vi "FR Estimate measurement time.vi"(11 "FFmeter settings":T1={"AC Source"={"AC Source type"=enum."Fluke 5XXX calibrator", "VISA"="", "Ref. clock (Hz)"=0.0, "status ref"=refnum}, "TWM pipe"="\\\\.\\pipe\\TWM:server", "Measurement status ref"=refnum, "TWM Status ref"=refnum, "Abort ref"=refnum, "DC meter"={"DC meter type"=enum."H/A/K 3458", "DC meter VISA"="", "NPLC"=10, "status ref"=refnum}, "FR Measurement properties"={"Measurement frequencies (Hz)"=[1000.0], "Sampling frequency (Hz)"=500000.0, "Signal amplitude (V)"=4.5, "AC-DC settle time (s)"=20.0, "Record length (multiples of period)"=[1000.0, 10000.0, 1000.0], "Measurement template file"=path "", "Row of START keyword"=1, "Row of STOP keyword"=0, "Calculate RMS from samples"=FALSE, "AC-DC warm up time (s)"=300.0, "Measurement template line"=[], "DC meter readings No."=10, "Algorithm"="TWM-WFFT", "Simultaneous measurement"=FALSE}, "Skip waiting ref"=refnum, "Octave paths"={"GNU Octave path"=path "C:/Program Files/GNU Octave/Octave-6.2.0/mingw64/bin", "TWM+QWTB path"=path "C:/Users/labina/Desktop/TWM-1.8.7.0-full/octprog", "lvlib path"=path "D:/martin/WAC/WACsw - github/control_software/Filter function meter/external libraries/GOLPI 0.7.3.1 source distribution LV 20.0 32 bit/lv_proc.dll"}, "FR Template definition"={"Keywords column"=0, "Sig. freq. column"=1, "Rec. len. column"=2, "Meas. points. row min to read"=9, "Meas. points. row max to read"=1509, "Properties column"=4, "Properties row start"=1, "Properties row end"=5, "Keyword START regexp"="", "Keyword STOP regexp"="", "HW data column"=7, "HW data row start"=1, "HW data row end"=3, "TIme and date column start"=3, "Digitizer value column start "=4, "DC mean column start "=6, "DC readings column start"=10}, "Recalculate-skip already calculated"=FALSE} {"FR Measurement properties"."Record length (multiples of period)" format="%#_3p"; "FR Measurement properties"."Sampling frequency (Hz)" format="%#_3p"; "FR Measurement properties"."Measurement frequencies (Hz)" format="%#_3p"}) -> (1 "Estimate as formatted text":string, 3 "Estimate of measurement time (s)":dbl)   [LabVIEW 2020]
doc: "Estimates the total measurement time based on the measurement settings and devices settings."
uses:
  FR GUI/Type definitions/FRmeter settings.ctl
  General AC source/Type definitions/AC Source.ctl
  General AC source/Type definitions/AC Source type.ctl
  General DC meter/Type definitions/DC meter.ctl
  General DC meter/Type definitions/DC meter type.ctl
  FR Measurement/Type definitions/FR Measuement properties.ctl
  Type definitions/FR Template definition.ctl
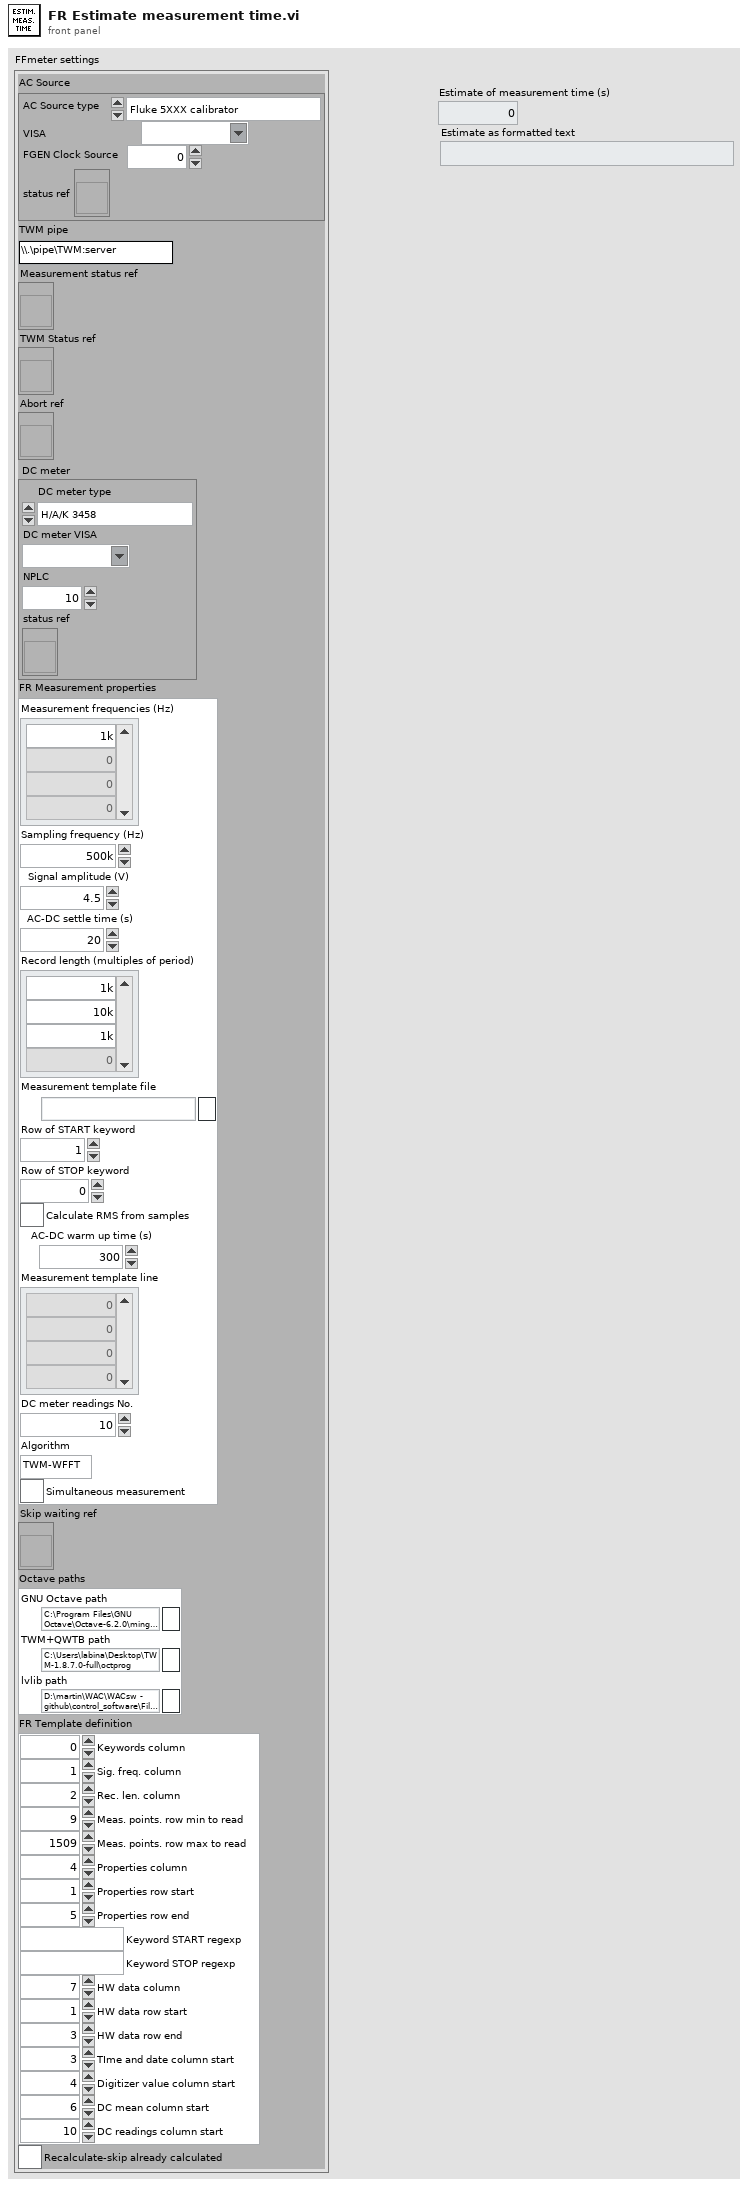
[diagram p1: front panel]
types:
  T1 = typedef "FRmeter settings.ctl" = cluster{"AC Source":T2, "TWM pipe":string, "Measurement status ref":refnum<vi>, "TWM Status ref":refnum<vi>, "Abort ref":refnum<vi>, "DC meter":T4, "FR Measurement properties":T6, "Skip waiting ref":refnum<vi>, "Octave paths":cluster{"GNU Octave path":path, "TWM+QWTB path":path, "lvlib path":path}, "FR Template definition":T7, "Recalculate-skip already calculated":bool}
  T2 = typedef "AC Source.ctl" = cluster{"AC Source type":T3, "VISA":refnum<visa-resource-name>, "Ref. clock (Hz)":dbl, "status ref":refnum<vi>}
  T3 = typedef "AC Source type.ctl" = enum16{"Fluke 5XXX calibrator", "Tektronix AFG3000 series", "dummy"}
  T4 = typedef "DC meter.ctl" = cluster{"DC meter type":T5, "DC meter VISA":refnum<visa-resource-name>, "NPLC":i32, "status ref":refnum<vi>}
  T5 = typedef "DC meter type.ctl" = enum16{"H/A/K 3458", "Fluke 8508A", "dummy", "Keithley 2182"}
  T6 = typedef "FR Measuement properties.ctl" = cluster{"Measurement frequencies (Hz)":dbl[], "Sampling frequency (Hz)":dbl, "Signal amplitude (V)":dbl, "AC-DC settle time (s)":dbl, "Record length (multiples of period)":dbl[], "Measurement template file":path, "Row of START keyword":i32, "Row of STOP keyword":i32, "Calculate RMS from samples":bool, "AC-DC warm up time (s)":dbl, "Measurement template line":i32[], "DC meter readings No.":i32, "Algorithm":string, "Simultaneous measurement":bool}
  T7 = typedef "FR Template definition.ctl" = cluster{"Keywords column":i32, "Sig. freq. column":i32, "Rec. len. column":i32, "Meas. points. row min to read":i32, "Meas. points. row max to read":i32, "Properties column":i32, "Properties row start":i32, "Properties row end":i32, "Keyword START regexp":string, "Keyword STOP regexp":string, "HW data column":i32, "HW data row start":i32, "HW data row end":i32, "TIme and date column start":i32, "Digitizer value column start ":i32, "DC mean column start ":i32, "DC readings column start":i32}
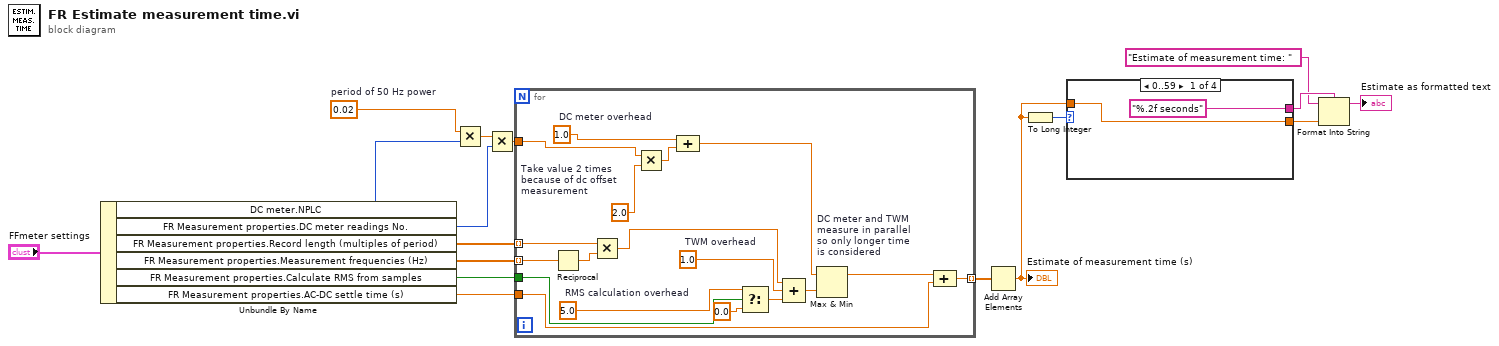
[diagram p0: block diagram]
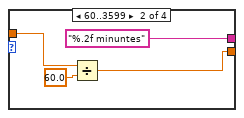
[diagram p2: hidden frame]
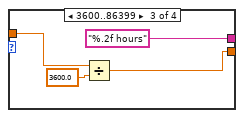
[diagram p3: hidden frame]
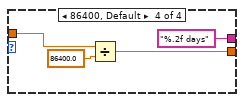
[diagram p4: hidden frame]
diagram:
  w15 = 0.02  # period of 50 Hz power
  n1 = Unbundle By Name("FFmeter settings") -> ("DC meter.NPLC"=w16:i32, "FR Measurement properties.DC meter readings No."=w14:i32, "FR Measurement properties.Record length (multiples of period)"=w11:dbl[], "FR Measurement properties.Measurement frequencies (Hz)"=w12:dbl[], "FR Measurement properties.Calculate RMS from samples"=w8:bool, "FR Measurement properties.AC-DC settle time (s)"=w2:dbl)
  n2 = Multiply(x=w15, y=w16) -> (x*y=w13:dbl)
  n3 = Multiply(x=w13, y=w14) -> (x*y=w10:dbl)
  n4 = for {
    tunnel: w12 -> [w35] mode=indexing
    tunnel: w11 -> [w33] mode=indexing
    tunnel: w10 -> [w20]
    tunnel: [w22] -> w9 mode=indexing
    tunnel: w8 -> [w29]
    tunnel: w2 -> [w23]
    w19 = 2.0  # Take value 2 times because of dc offset measurement
    w21 = 1.0  # DC meter overhead
    w28 = 5.0  # RMS calculation overhead
    w32 = 1.0  # TWM overhead
    n5 = Reciprocal(x=w35) -> (1/x=w34:dbl)
    n6 = Multiply(x=w33, y=w34) -> (x*y=w31:dbl)
    n7 = Multiply(x=w20, y=w19) -> (x*y=w18:dbl)
    n8 = Compound Arithmetic op=unknown(w21, w18) -> (w25:dbl)
    n9 = Select(t=w28, s=w29, f=0.0 ("RMS calculation overhead")) -> (s? t:f=w26:dbl)
    n10 = Compound Arithmetic op=ADD(w31, w32, w26) -> (w30:dbl)
    n11 = Max & Min "DC meter and TWM\nmeasure in parallel\nso only longer time\nis considered"(x=w25, y=w30) -> (max(x,y)=w24:dbl)  [unwired: 1 out]
    n12 = Compound Arithmetic op=ADD(w24, w23) -> (w22:dbl)
  }
  n13 = Add Array Elements(numeric array=w9) -> (sum=w1:dbl)
  "Estimate of measurement time (s)" <- w1
  n14 = To Long Integer(number=w1) -> (32bit integer=w7:i32)
  n15 = case shown="0..59" w7 {
    tunnel: w1 -> [w36 w40 w44 w48]
    tunnel: [w36 w38 w43 w47] -> w6
    tunnel: ["%.2f seconds" ("format string") "%.2f minuntes" ("format string") "%.2f hours" ("format string") "%.2f days" ("format string")] -> w5
    frame 0..59 {
    }
    frame 60..3599 {
      n16 = Divide(x=w40, y=60.0) -> (x/y=w38:dbl)
    }
    frame 3600..86399 {
      n17 = Divide(x=w44, y=3600.0) -> (x/y=w43:dbl)
    }
    frame 86400, Default {
      n18 = Divide(x=w48, y=86400.0) -> (x/y=w47:dbl)
    }
  }
  n19 = Format Into String(format string=w5, initial string="Estimate of measurement time: ", w6) -> (resulting string=→"Estimate as formatted text":string)  [unwired: 1 in, 1 out]
